vi "Device in Stack.vi"(8 "error in (no error)":errorcluster, 9 "Device UID":string, 11 "IP Connection in":refnum<class "IP Connection.lvclass">) -> (0 "error out":errorcluster, 1 "Device already in Stack":bool, 3 "IP Connection out":refnum<class "IP Connection.lvclass">)   [LabVIEW 2011, in "Tinkerforge.lvlib" / "IP Connection.lvclass"]
doc: "This VI checks if the <B>Device UID</B> is already in the registered stack."
uses:
  IP Connection.lvclass
  Device/Device.lvclass
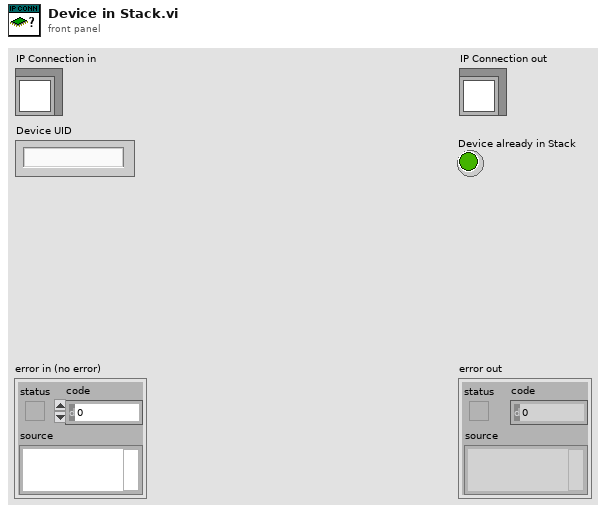
[diagram p1: front panel]
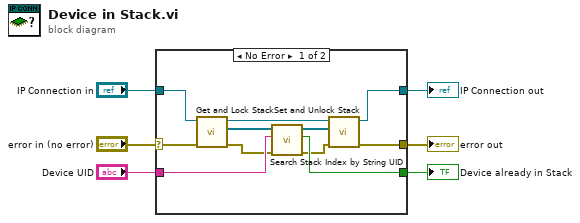
[diagram p0: block diagram]
diagram:
  n1 = case shown="No Error" "error in (no error)" {
    selector: "error in (no error)" -> [w9 w19]
    tunnel: [w14 w19] -> w5
    tunnel: [w12 w18] -> w3
    tunnel: "IP Connection in" -> [w13 w18]
    tunnel: "Device UID" -> [w17 _]
    tunnel: [w16 _] -> w1
    frame No Error {
      n2 = call "Get and Lock Stack.vi"("error in (no error)"=w9, "IP Connection in"=w13) -> ("error out"=w7:errorcluster, "Stack"=w10:refnum<class "Device.lvclass">[], "IP Connection out"=w15:refnum<class "IP Connection.lvclass">)  [unwired: 7 in]
      n3 = call "Search Stack Index by String UID.vi"("error in (no error)"=w7, "Device UID"=w17, "Stack in"=w10) -> ("error out"=w8:errorcluster, "Device found?"=w16:bool, "Stack out"=w11:refnum<class "Device.lvclass">[])  [unwired: 4 in, 2 out]
      n4 = call "Set and Unlock Stack.vi"("error in (no error)"=w8, "Stack"=w11, "IP Connection in"=w15) -> ("error out"=w14:errorcluster, "IP Connection out"=w12:refnum<class "IP Connection.lvclass">)  [unwired: 7 in]
    }
    frame Error {
    }
  }
  "error out" <- w5
  "IP Connection out" <- w3
  "Device already in Stack" <- w1
